vi "Start Actor.vi"() -> ()   [LabVIEW 2012, in "CS++Core-Examples.lvlib"]
doc: "This example illustrates how to start an actor via Factory and to send an Stop-Message on stop."
uses:
  CS++Core-Examples.lvlib
  Core/Classes/CS++BaseClasses/Factory/CS++Factory.lvclass
  Core/Classes/CS++BaseClasses/Factory/CS++Factory.lvclass/CS++Factory.ctl
  <vilib>/ActorFramework/Message Queue/Message Queue.lvclass/Message Queue.ctl
  <vilib>/ActorFramework/Message Enqueuer/Message Enqueuer.lvclass/Message Enqueuer.ctl
  <vilib>/ActorFramework/Message Enqueuer/Enqueue.vi
  <vilib>/ActorFramework/Message Priority Queue/Priority Enqueue.vi
  <vilib>/ActorFramework/Stop Msg/Stop Msg.lvclass
  <vilib>/ActorFramework/Actor/Actor.lvclass
  <vilib>/ActorFramework/Message Queue/Message Queue.lvclass
panel:
  in  "Configuration File":path=path "C:/User/Brand/Git/CSPP/Core/CS++Example.ini"
  in  "Stop Button":bool
  in  "Object Name":string
  out "Attributes found?":bool
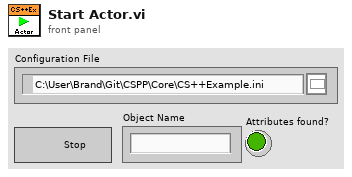
[diagram p1: front panel]
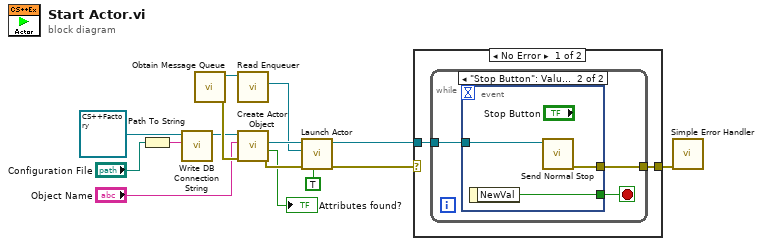
[diagram p0: block diagram]
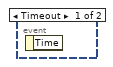
[diagram p2: hidden frame]
diagram:
  n1 = Path To String(path="Configuration File") -> (string=w2:string)
  n2 = call "Write DB Connection String.vi"("DB Connection String"=w2, "CS++Factory in"=refnum<class "CS++Factory.lvclass"> refnum ("CS++BaseClasses.lvlib:CS++Factory.lvclass")) -> ("CS++Factory out"=w3:refnum<class "CS++Factory.lvclass">)  [unwired: 8 in, 1 out]
  n3 = call <vilib>:"Obtain Message Queue.vi"() -> ("error out"=w14:errorcluster, "Message Queue"=w15:refnum<class "Message Queue.lvclass">)  [unwired: 10 in]
  n4 = call <vilib>:"Read Enqueuer.vi"("Message Queue"=w15) -> ("Message Enqueuer"=w12:refnum<class "Message Enqueuer.lvclass">)  [unwired: 10 in]
  n5 = call "Create Actor Object.vi"("error in (no error)"=w14, "Object Name"="Object Name", "CS++Factory in"=w3) -> ("error out"=w11:errorcluster, "Attributes found?"=→"Attributes found?":bool, "C++BaseActor"=w13:refnum<class "CS++BaseActor.lvclass">)  [unwired: 5 in, 1 out]
  n6 = call <vilib>:"Launch Actor.vi"("Open Actor Core front panel? (F)"=TRUE, "error in (no error)"=w11, "Actor-to-Caller Enqueuer"=w12, "Actor"=w13) -> ("error out"=w7:errorcluster, "Caller-To-Actor Enqueuer"=w8:refnum<class "Message Enqueuer.lvclass">)  [unwired: 6 in]
  n7 = case shown="No Error" w7 {
    selector: w7 -> [_ w24]
    tunnel: w8 -> [w17 _]
    tunnel: [w16 w24] -> w6
    frame No Error {
      n8 = while {
        tunnel: w17 -> [w19]
        tunnel: [w18] -> w16
        stop <- w20 stop-if-true
        n9 = event shown="[1] \"Stop Button\": Value Change" {
          selector: _ -> [_ _]
          dyn-events: _ -> [_ _]
          timeout: _ -> [_ _]
          tunnel: [_ w23] -> w20
          tunnel: w19 -> [_ w22]
          tunnel: [_ w21] -> w18
          event Timeout {
            n10 = event-data() -> ()  [unwired: 1 in, 1 out]
          }
          event "Stop Button": Value Change {
            n11 = event-data() -> ("NewVal"=w23:bool)  [unwired: 1 in]
            n12 = call <vilib>:"Send Normal Stop.vi"("Message Enqueuer"=w22) -> ("error out"=w21:errorcluster)  [unwired: 10 in]
          }
        }
      }
    }
    frame Error {
    }
  }
  n13 = call <vilib>:"Simple Error Handler.vi"("error in (no error)"=w6) -> ()  [unwired: 4 in, 5 out]
